vi "close.vi"(8 "error in":errorcluster, 11 "SystemLin Tag Module runtime in":refnum<class "SystemLink File runtime.lvclass">) -> (0 "error out":errorcluster)   [LabVIEW 2015, in "SystemLink File runtime.lvclass"]
doc: "Provides an interface for terminating a module instance. While this interface performs no operations, a child should close and deallocate any open references or memory."
uses:
  SystemLink File runtime.lvclass
  SystemLink File runtime.lvclass/SystemLink File runtime.ctl
  <vilib>/Skyline/Configuration/Configuration_class/NI Skyline Configuration.lvclass
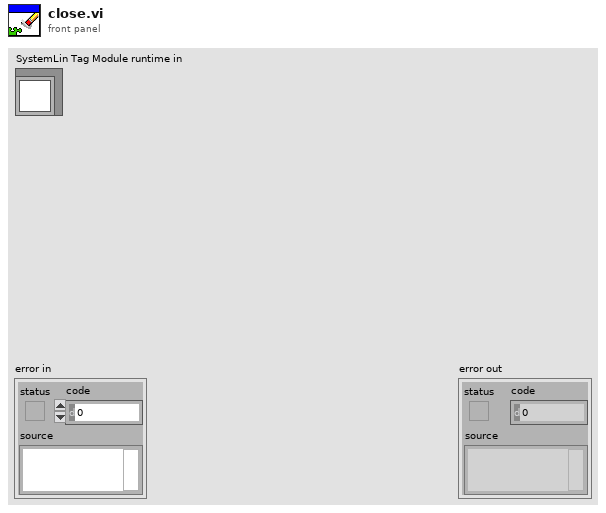
[diagram p1: front panel]
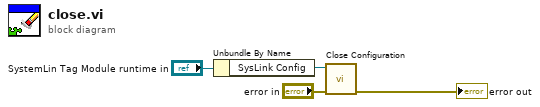
[diagram p0: block diagram]
diagram:
  n1 = Unbundle By Name("SystemLin Tag Module runtime in") -> ("SysLink Config"=w2:refnum<class "NI Skyline Configuration.lvclass">)
  n2 = call-dynamic "Close Configuration.vi"("error in (no error)"="error in", "configuration in"=w2) -> ("error out"=→"error out":errorcluster)  [unwired: 9 in]
